vi "Start Testing.vi"(8 "error in (no error)":errorcluster, 9 "Test Settings":T1, 10 "Model in":refnum<class "Model.lvclass">, 11 "Wait For User Input State in":refnum<class "Wait For User Input State.lvclass">) -> (0 "error out":errorcluster, 2 "Model out":refnum<class "Model.lvclass">, 3 "Wait For User Input State out":refnum<class "Wait For User Input State.lvclass">)   [LabVIEW 2016, in "Wait For User Input State.lvclass"]
uses:
  Wait For User Input State.lvclass
  Model/Model/Model.lvclass
  Typedefs/TestSettings.ctl
  Typedefs/StateTypes.ctl
  Model/Model/Model.lvclass/Model.ctl
  Typedefs/M1M3SupportEUI_TypeDefs.lvlib
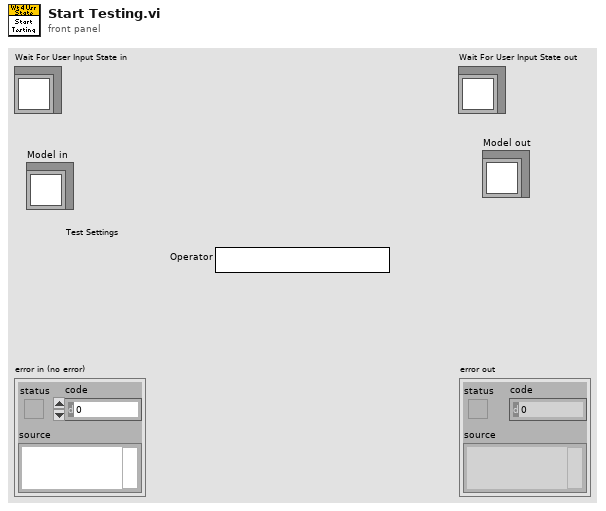
[diagram p1: front panel]
types:
  T1 = typedef "M1M3SupportEUI_TypeDefs.lvlib/TestSettings.ctl" = cluster{"Operator":string}
  T2 = typedef "M1M3SupportEUI_TypeDefs.lvlib/StateTypes.ctl" = enum16{"Offline State", "Fault State", "Standby State", "Disabled State", "Enabled State", "Wait For User Input State", "Test Actuator State"}
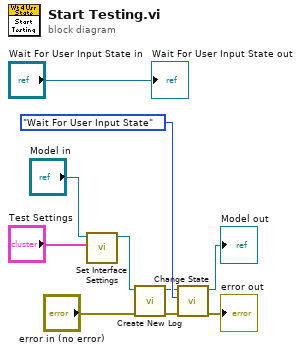
[diagram p0: block diagram]
diagram:
  n1 = call "Set Interface Settings.vi"("Interface Settings"="Test Settings", "Model in"="Model in") -> ("Model out"=w4:refnum<class "Model.lvclass">)  [unwired: 9 in]
  n2 = call "Create New Log.vi"("error in (no error)"="error in (no error)", "Model in"=w4) -> ("error out"=w2:errorcluster, "Model out"=w1:refnum<class "Model.lvclass">)  [unwired: 8 in]
  n3 = call "Change State.vi"("error in (no error)"=w2, "State Types"=StateTypes."Wait For User Input State" ("State:"), "Model in"=w1) -> ("error out"=→"error out":errorcluster, "Model out"=→"Model out":refnum<class "Model.lvclass">)  [unwired: 7 in]
  "Wait For User Input State out" <- "Wait For User Input State in"
